vi "例程49-生产与消费者设计模式.vi"() -> ()   [LabVIEW 2016]
doc: "该模板用于创建生产者／消费者模式的应用程序，以事件驱动的方式，生成队列中的项。如需通过响应事件实现代码的异步执行，同时不影响用户界面的响应速度，可考虑用该模式替代“用户界面事件处理器”模式。"
panel:
  in  "新事件":bool caption="元素入队列"
  out "数据（可为任意类型）":string
  in  "Enqueue Element":bool caption="元素入队列"
  in  "stop":bool caption="停止"
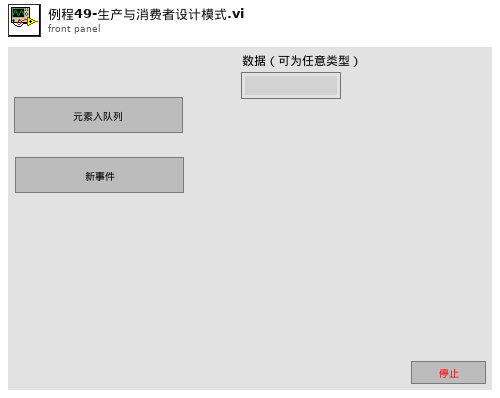
[diagram p1: front panel]
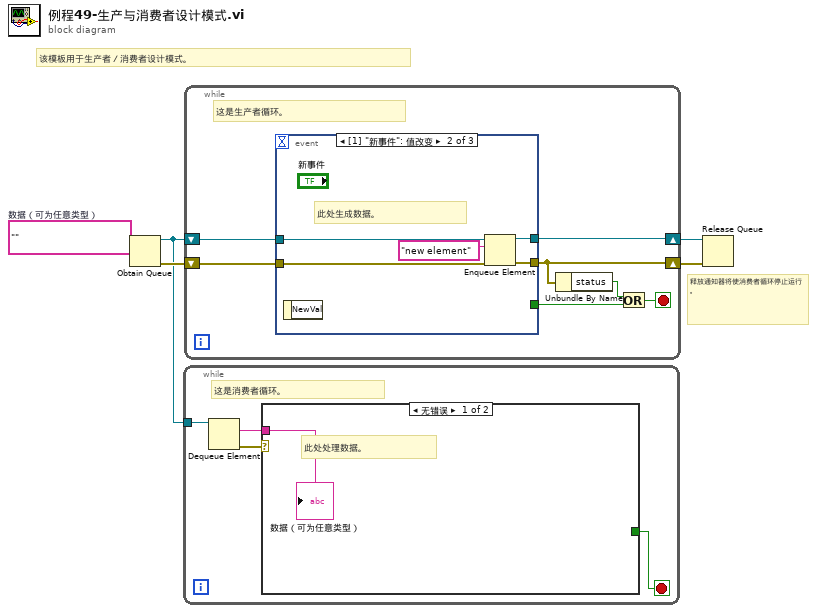
[diagram p0: block diagram]
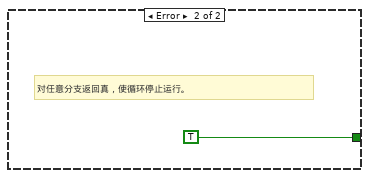
[diagram p2: hidden frame]
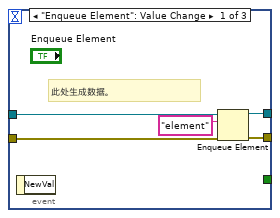
[diagram p3: hidden frame]
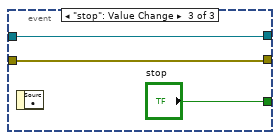
[diagram p4: hidden frame]
diagram:
  w3 = ""  # 数据（可为任意类型）
  # "释放通知器将使消费者循环停止运行。"
  # "该模板用于生产者／消费者设计模式。"
  n1 = Obtain Queue(element data type=w3) -> (queue out=w2:refnum<queue>, error out=w5:errorcluster)  [unwired: 4 in, 1 out]
  n2 = while {
    tunnel: w2 -> [w9]
    stop <- w6 stop-if-true
    # "这是消费者循环。"
    n3 = Dequeue Element(queue=w9) -> (element=w7:string, error out=w8:errorcluster)  [unwired: 2 in, 2 out]
    n4 = case shown="无错误" w8 {
      tunnel: w7 -> [w10 _]
      tunnel: [_ TRUE] -> w6
      frame No Error {
        # "此处处理数据。"
        "数据（可为任意类型）" <- w10
      }
      frame Error {
        # "对任意分支返回真，使循环停止运行。"
      }
    }
  }
  n5 = while {
    shift-right: [w14] -> w4
    shift-left: w5 -> [w17]
    shift-right: [w12] -> w1
    shift-left: w2 -> [w18]
    stop <- w15 stop-if-true
    # "这是生产者循环。"
    n6 = event shown="[1] \"新事件\": 值改变" {
      selector: _ -> [_ _ _]
      dyn-events: _ -> [_ _ _]
      timeout: _ -> [_ _ _]
      tunnel: w18 -> [w23 w28 w29]
      tunnel: w17 -> [w22 w27 w30]
      tunnel: [w21 w26 w30] -> w14
      tunnel: [_ _ "stop"] -> w16
      tunnel: [w19 w24 w29] -> w12
      event "Enqueue Element": Value Change {
        # "此处生成数据。"
        n7 = event-data() -> ()  [unwired: 1 in, 1 out]
        n8 = Enqueue Element(queue=w23, element="element", error in (no error)=w22) -> (queue out=w19:refnum<queue>, error out=w21:errorcluster)  [unwired: 1 in, 1 out]
      }
      event "新事件": Value Change {
        # "此处生成数据。"
        n9 = event-data() -> ()  [unwired: 1 in, 1 out]
        n10 = Enqueue Element(queue=w28, element="new element", error in (no error)=w27) -> (queue out=w24:refnum<queue>, error out=w26:errorcluster)  [unwired: 1 in, 1 out]
      }
      event "stop": Value Change {
        n11 = event-data() -> ()  [unwired: 1 in, 1 out]
      }
    }
    n12 = Unbundle By Name(w14) -> ("status"=w13:bool)
    n13 = Or(x=w13, y=w16) -> (x .or. y?=w15:bool)
  }
  n14 = Release Queue(queue=w1, error in (no error)=w4) -> ()  [unwired: 1 in, 3 out]
